vi "goToNode.vi"(8 "error in (no error)":errorcluster, 10 "Node Path":string, 11 "xceNode in":refnum<class "xceNode.lvclass">) -> (0 "error out":errorcluster, 2 "goToNode* out":refnum<data-value>, 3 "xceNode out":refnum<class "xceNode.lvclass">)   [LabVIEW 2013, in "xceNode.lvclass"]
doc: "Navigates to a node in the tree data structure, give the nodes path. Node path is a '\\' deliminated string (for example Node0\\Node2\\Node5).\n\nTypically this path is formed from a tree control with a little manipulation."
uses:
  xceNode.lvclass
  xceNode.lvclass/xceNode.ctl
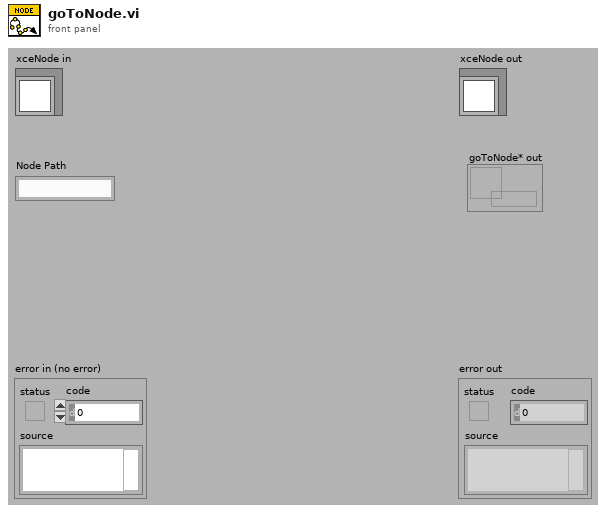
[diagram p1: front panel]
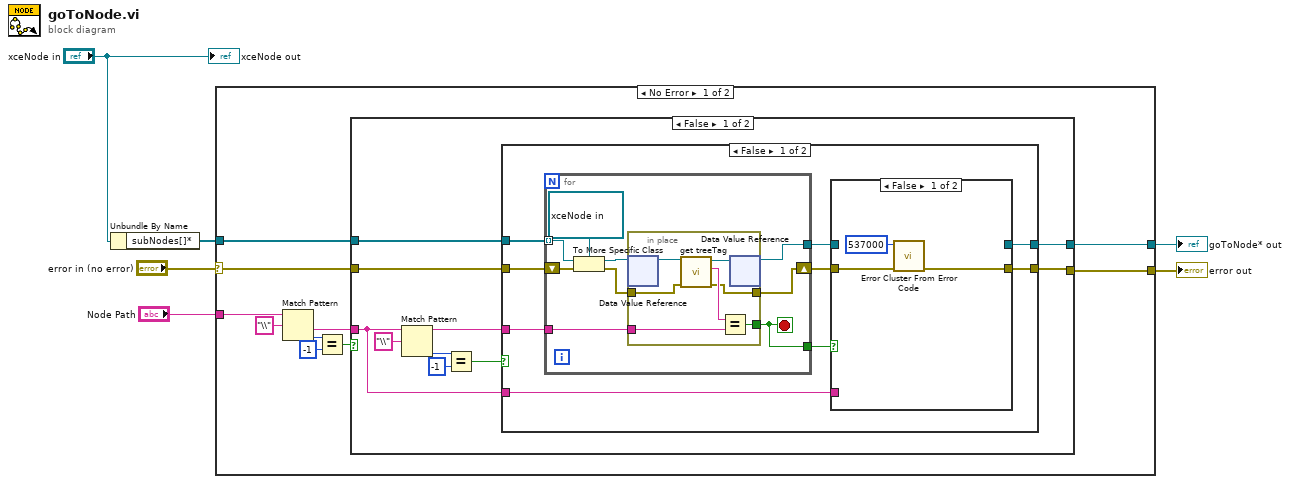
[diagram p0: block diagram]
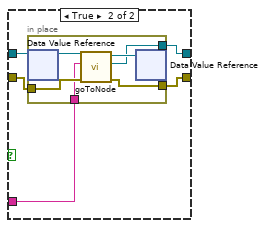
[diagram p2: hidden frame]
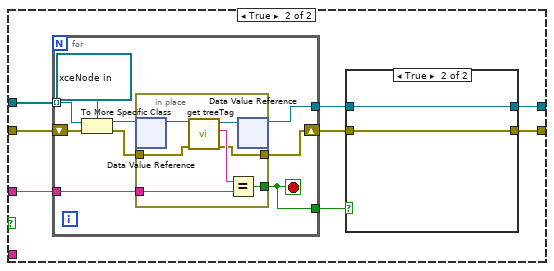
[diagram p3: hidden frame]
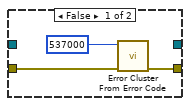
[diagram p4: hidden frame]
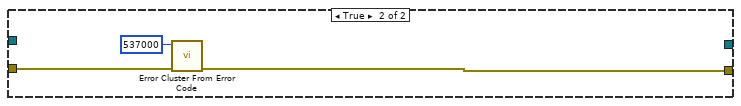
[diagram p5: hidden frame]
diagram:
  n1 = Unbundle By Name("xceNode in") -> ("subNodes[]*"=w3:refnum<data-value>[])
  n2 = case shown="No Error" "error in (no error)" {
    selector: "error in (no error)" -> [w11 w98]
    tunnel: [w10 w98] -> w5
    tunnel: "Node Path" -> [w16 _]
    tunnel: w3 -> [w8 _]
    tunnel: [w7 _] -> w1
    frame No Error {
      n3 = Match Pattern(string=w16, regular expression="\\") -> (after substring=w9:string, offset past match=w14:i32)  [unwired: 1 in, 2 out]
      n4 = Equal?(x=w14, y=-1) -> (x = y?=w12:bool)
      n5 = case shown="False" w12 {
        tunnel: w11 -> [w21 w96]
        tunnel: [w19 w95] -> w10
        tunnel: w9 -> [w17 _]
        tunnel: w8 -> [w20 _]
        tunnel: [w18 _] -> w7
        frame False {
          n6 = Match Pattern(string=w17, regular expression="\\") -> (before substring=w22:string, offset past match=w24:i32)  [unwired: 1 in, 2 out]
          n7 = Equal?(x=w24, y=-1) -> (x = y?=w23:bool)
          n8 = case shown="False" w23 {
            tunnel: w22 -> [w33 w71]
            tunnel: w20 -> [w35 w73]
            tunnel: w21 -> [w34 w72]
            tunnel: [w29 w67] -> w19
            tunnel: [w30 w66] -> w18
            tunnel: w17 -> [w28 _]
            frame False {
              n9 = for {
                tunnel: w35 -> [w58] mode=indexing
                tunnel: w33 -> [w54]
                tunnel: [w53] -> w27
                shift-right: [w51] -> w31
                shift-left: w34 -> [w57]
                tunnel: [w50] -> w32
                stop <- w53 stop-if-true
                n10 = To More Specific Class(target class=refnum<data-value> refnum ("data value reference"), reference=w58, error in=w57) -> (specific class reference=w55:refnum<data-value>, error out=w52:errorcluster)
                n11 = in-place {
                  in-place-border: w54 -> [w63]
                  in-place-border: [w61] -> w53
                  in-place-border: w52 -> [w60]
                  in-place-border: [w59] -> w51
                  n12 = in-place-dvr #1(w55) -> (w65:refnum<class "xceNode.lvclass">)  [unwired: 1 out]
                  n13 = call "get treeTag.vi"("error in (no error)"=w60, "xceNode in"=w65) -> ("error out"=w59:errorcluster, "treeTag"=w62:string, "xceNode out"=w64:refnum<class "xceNode.lvclass">)  [unwired: 7 in]
                  n14 = Equal?(x=w62, y=w63) -> (x = y?=w61:bool)
                  n15 = in-place-dvr #1(w64) -> (w50:refnum<data-value>)  [unwired: 1 out]
                }
              }
              n16 = case shown="False" w27 {
                tunnel: w32 -> [_ w43]
                tunnel: w31 -> [w37 w41]
                tunnel: [w36 w40] -> w29
                tunnel: [_ w42] -> w30
                tunnel: w28 -> [_ w39]
                frame False {
                  n17 = call <vilib>:"Error Cluster From Error Code.vi"("error in (no error)"=w37, "error code (0)"=537000) -> ("error out"=w36:errorcluster)  [unwired: 7 in]
                }
                frame True {
                  n18 = in-place {
                    in-place-border: [w47] -> w42
                    in-place-border: w41 -> [w46]
                    in-place-border: [w45] -> w40
                    in-place-border: w39 -> [w44]
                    n19 = in-place-dvr #2(w43) -> (w49:refnum<class "xceNode.lvclass">)  [unwired: 1 out]
                    n20 = call "goToNode.vi"("error in (no error)"=w46, "Node Path"=w44, "xceNode in"=w49) -> ("error out"=w45:errorcluster, "goToNode* out"=w47:refnum<data-value>, "xceNode out"=w48:refnum<class "xceNode.lvclass">)  [unwired: 6 in]
                    n21 = in-place-dvr #2(w48) -> ()  [unwired: 2 out]
                  }
                }
              }
            }
            frame True {
              n22 = for {
                tunnel: w73 -> [w87] mode=indexing
                tunnel: w71 -> [w83]
                tunnel: [w82] -> w70
                shift-right: [w80] -> w68
                shift-left: w72 -> [w86]
                tunnel: [w79] -> w69
                stop <- w82 stop-if-true
                n23 = To More Specific Class(target class=refnum<data-value> refnum ("data value reference"), reference=w87, error in=w86) -> (specific class reference=w84:refnum<data-value>, error out=w81:errorcluster)
                n24 = in-place {
                  in-place-border: w83 -> [w92]
                  in-place-border: [w90] -> w82
                  in-place-border: w81 -> [w89]
                  in-place-border: [w88] -> w80
                  n25 = in-place-dvr #3(w84) -> (w94:refnum<class "xceNode.lvclass">)  [unwired: 1 out]
                  n26 = call "get treeTag.vi"("error in (no error)"=w89, "xceNode in"=w94) -> ("error out"=w88:errorcluster, "treeTag"=w91:string, "xceNode out"=w93:refnum<class "xceNode.lvclass">)  [unwired: 7 in]
                  n27 = Equal?(x=w91, y=w92) -> (x = y?=w90:bool)
                  n28 = in-place-dvr #3(w93) -> (w79:refnum<data-value>)  [unwired: 1 out]
                }
              }
              n29 = case shown="True" w70 {
                tunnel: w69 -> [_ w77]
                tunnel: w68 -> [w74 w78]
                tunnel: [w76 w78] -> w67
                tunnel: [_ w77] -> w66
                frame False {
                  n30 = call <vilib>:"Error Cluster From Error Code.vi"("error in (no error)"=w74, "error code (0)"=537000) -> ("error out"=w76:errorcluster)  [unwired: 7 in]
                }
                frame True {
                }
              }
            }
          }
        }
        frame True {
          n31 = call <vilib>:"Error Cluster From Error Code.vi"("error in (no error)"=w96, "error code (0)"=537000) -> ("error out"=w95:errorcluster)  [unwired: 7 in]
        }
      }
    }
    frame Error {
    }
  }
  "error out" <- w5
  "goToNode* out" <- w1
  "xceNode out" <- "xceNode in"
